vi "Exo3.vi"() -> ()   [LabVIEW 2018]
panel:
  out "Résidus":bool
  out "Nom":string
  out "Prénom":string
  in  "Nom Brut":string
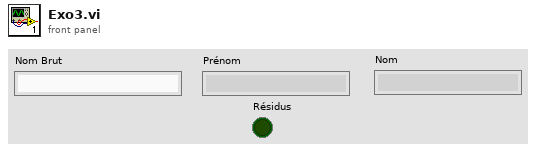
[diagram p1: front panel]
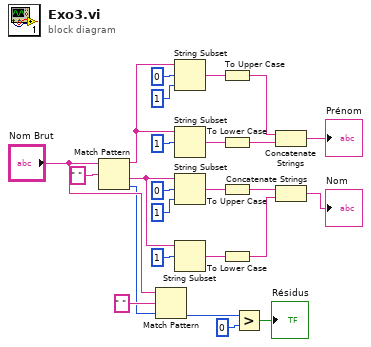
[diagram p0: block diagram]
diagram:
  n1 = Match Pattern(string="Nom Brut", regular expression=" ") -> (before substring=w13:string, after substring=w1:string, offset past match=w20:i32)  [unwired: 1 in, 1 out]
  n2 = Match Pattern(string="Nom Brut", regular expression=" ", offset (0)=w20) -> (offset past match=w19:i32)  [unwired: 3 out]
  n3 = String Subset(string=w13, offset (0)=0, length (rest)=1 ("length (rest)")) -> (substring=w16:string)
  n4 = String Subset(string=w13, offset (0)=1) -> (substring=w11:string)  [unwired: 1 in]
  n5 = String Subset(string=w1, offset (0)=0, length (rest)=1 ("length (rest)")) -> (substring=w7:string)
  n6 = String Subset(string=w1, offset (0)=1) -> (substring=w4:string)  [unwired: 1 in]
  n7 = To Upper Case(1:w16) -> (0:w15:string)
  n8 = To Lower Case(string=w11) -> (all lower case string=w10:string)
  n9 = To Upper Case(1:w7) -> (0:w6:string)
  n10 = To Lower Case(string=w4) -> (all lower case string=w3:string)
  n11 = Greater?(x=w19, y=0) -> (0:→"Résidus":bool)
  n12 = Concatenate Strings(w15, w10) -> (→"Prénom":string)
  n13 = Concatenate Strings(w6, w3) -> (→"Nom":string)
